vi "move in wave.vi"(8 "error in (no error)":errorcluster, 9 "Wave Specs":T2={"XAmp"=0.0, "YAmp"=0.0, "Zamp"=0.0, "T (sec)"=10.0, "Wave Type"=enum."Sine"}, 10 "output wave?":bool=TRUE, 11 "ASI stage":T1) -> (0 "error out":errorcluster, 3 "ASI stage out":T1)   [LabVIEW 2010]
uses:
  stage properties.ctl
  <vilib>/ptbypt/NI_PtbyPt.lvlib
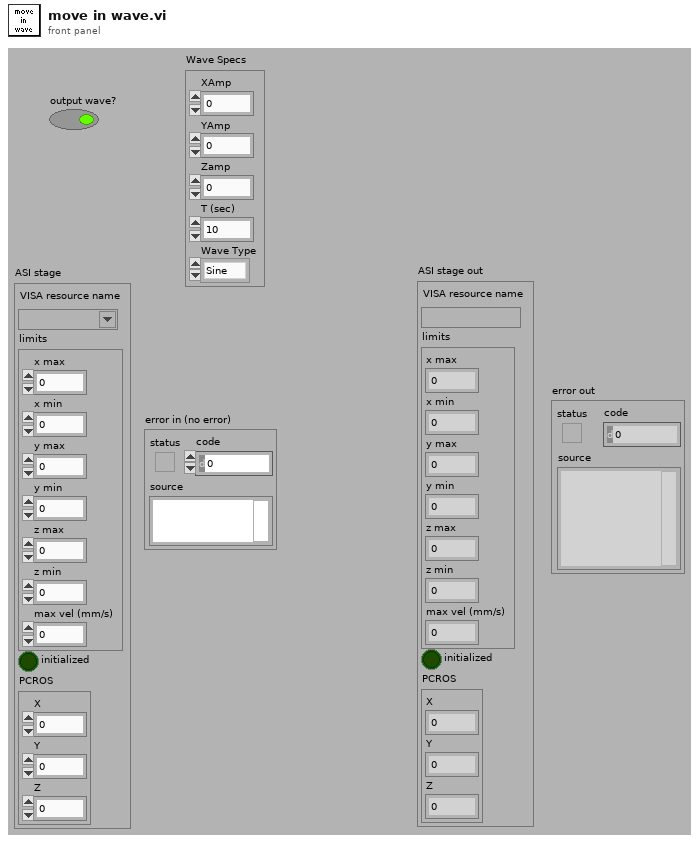
[diagram p1: front panel]
types:
  T1 = typedef "stage properties.ctl" = cluster{"VISA resource name":refnum<visa-resource-name>, "limits":cluster{"x max":dbl, "x min":dbl, "y max":dbl, "y min":dbl, "z max":dbl, "z min":dbl, "max vel (mm/s)":dbl}, "initialized":bool, "PCROS":cluster{"X":dbl, "Y":dbl, "Z":dbl}}
  T2 = cluster{"XAmp":dbl, "YAmp":dbl, "Zamp":dbl, "T (sec)":dbl, "Wave Type":enum16{"Sine", "Triange"}}
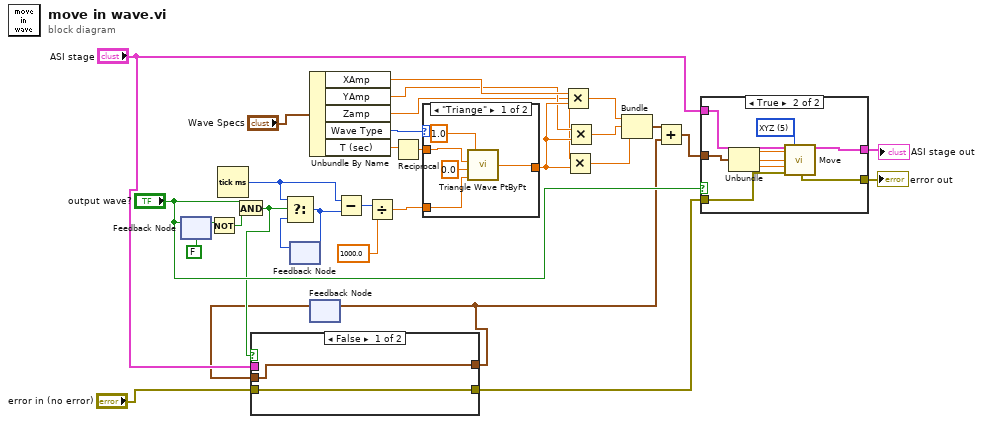
[diagram p0: block diagram]
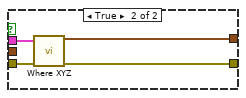
[diagram p2: hidden frame]
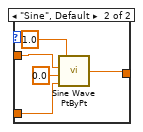
[diagram p4: hidden frame]
diagram:
  n1 = feedback-in #1("output wave?") -> ()
  n2 = feedback #1(FALSE ("output wave?")) -> (w31:bool)
  n3 = Not(x=w31) -> (.not. x?=w30:bool)
  n4 = Tick Count (ms)() -> (millisecond timer value=w28:u32)
  n5 = And(x="output wave?", y=w30) -> (x .and. y?=w12:bool)
  n6 = feedback #2() -> (w29:u32)  [unwired: 1 in]
  n7 = Select(t=w28, s=w12, f=w29) -> (s? t:f=w27:u32)
  n8 = feedback-in #2(w27) -> ()
  n9 = Unbundle By Name("Wave Specs") -> ("XAmp"=w18:dbl, "YAmp"=w17:dbl, "Zamp"=w16:dbl, "Wave Type"=w23:enum16{"Sine", "Triange"}, "T (sec)"=w22:dbl)
  n10 = feedback #3() -> (w8:cluster{"X out":dbl, "Y out":dbl, "Z out":dbl})  [unwired: 1 in]
  n11 = case shown="False" w12 {
    tunnel: "error in (no error)" -> [w33 w37]
    tunnel: "ASI stage" -> [_ w36]
    tunnel: [w33 w35] -> w9
    tunnel: [w32 w34] -> w3
    tunnel: w8 -> [w32 _]
    frame False {
    }
    frame True {
      n12 = call "Where XYZ.vi"("ASI stage"=w36, "error in (no error)"=w37) -> ("location"=w34:cluster{"X out":dbl, "Y out":dbl, "Z out":dbl}, "error out"=w35:errorcluster)  [unwired: 11 in, 1 out]
    }
  }
  n13 = feedback-in #3(w3) -> ()
  n14 = Subtract(x=w28, y=w27) -> (x-y=w26:u32)
  n15 = Divide(x=w26, y=1000.0) -> (x/y=w20:dbl)
  n16 = Reciprocal(x=w22) -> (1/x=w21:dbl)
  n17 = case shown="\"Triange\"" w23 {
    tunnel: w21 -> [w42 w47]
    tunnel: w20 -> [w40 w45]
    tunnel: [w38 w43] -> w19
    frame "Triange" {
      n18 = call <vilib>:"Triangle Wave PtByPt.vi"("time"=w40, "phase"=0.0, "frequency"=w42, "amplitude"=1.0) -> ("triangle wave"=w38:dbl)
    }
    frame "Sine", Default {
      n19 = call <vilib>:"Sine Wave PtByPt.vi"("time"=w45, "phase"=0.0, "frequency"=w47, "amplitude"=1.0) -> ("sine wave"=w43:dbl)
    }
  }
  n20 = Multiply(x=w18, y=w19) -> (x*y=w7:dbl)
  n21 = Multiply(x=w16, y=w19) -> (x*y=w5:dbl)
  n22 = Multiply(x=w17, y=w19) -> (x*y=w6:dbl)
  n23 = Bundle(w7, w6, w5) -> (w4:cluster{dbl, dbl, dbl})  [unwired: 1 in]
  n24 = Add(x=w4, y=w3) -> (x+y=w2:cluster{dbl, dbl, dbl})
  n25 = case shown="True" "output wave?" {
    tunnel: "ASI stage" -> [w49 w57]
    tunnel: w9 -> [w48 w56]
    tunnel: [w48 w55] -> w14
    tunnel: [w49 w54] -> w13
    tunnel: w2 -> [_ w53]
    frame False {
    }
    frame True {
      w58 = u16 5 items=["No axis", "X", "Y", "Z", "XY", "XYZ"] ("Axis configuration")
      n26 = Unbundle(w53) -> (w52:dbl, w51:dbl, w50:dbl)
      n27 = call "Move.vi"("ASI stage"=w57, "Axis configuration"=w58, "x"=w52, "y"=w51, "z"=w50, "error in (no error)"=w56) -> ("ASI stage out"=w54:T1, "error out"=w55:errorcluster)  [unwired: 8 in]
    }
  }
  "ASI stage out" <- w13
  "error out" <- w14
